vi "SetPosition.vi"(8 "error in (no error)":errorcluster, 10 "Position":T1, 11 "3D Scene in":refnum<class "3D Scene.lvclass">) -> (0 "error out":errorcluster, 3 "3D Scene out":refnum<class "3D Scene.lvclass">)   [LabVIEW 2015, in "3D Scene.lvclass"]
uses:
  3D Scene.lvclass
  <vilib>/Utility/miscctls.llb/LV3DPointTypeDef.ctl
  3D Scene.lvclass/3D Scene.ctl
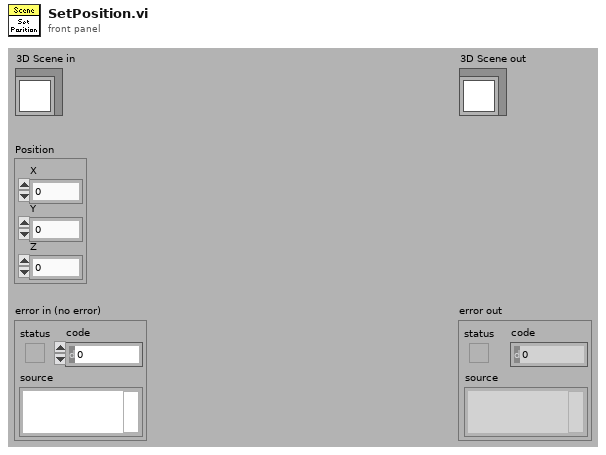
[diagram p1: front panel]
types:
  T1 = typedef "LV3DPointTypeDef.ctl" = cluster{"X":sgl, "Y":sgl, "Z":sgl}
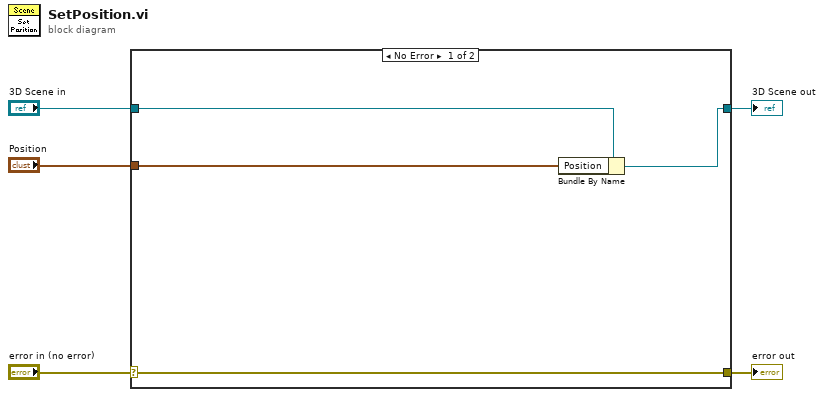
[diagram p0: block diagram]
diagram:
  n1 = case shown="No Error" "error in (no error)" {
    selector: "error in (no error)" -> [w7 w11]
    tunnel: [w7 w11] -> w4
    tunnel: [w6 w10] -> w2
    tunnel: "3D Scene in" -> [w9 w10]
    tunnel: "Position" -> [w8 _]
    frame No Error {
      n2 = Bundle By Name(cluster=w9, "Position"=w8) -> (w6:refnum<class "3D Scene.lvclass">)
    }
    frame Error {
    }
  }
  "error out" <- w4
  "3D Scene out" <- w2
